vi "readFromXML.vi"(8 "error in (no error)":errorcluster, 10 "XML in":string, 11 "CableWrapCommands in":refnum<class "CableWrapCommands.lvclass">) -> (0 "error out":errorcluster, 3 "CableWrapCommands out":refnum<class "CableWrapCommands.lvclass">)   [LabVIEW 2014, in "TCSDataDefinitions.lvlib" / "TCSCommand.lvlib" / "CableWrapCommands.lvlib" / "CableWrapCommands.lvclass"]
uses:
  CableWrapCommands.lvclass
  CableWrapCommands.lvclass/CableWrapCommands.ctl
  TCSTcsCommand/TCSTcsCommand.lvclass
  <userlib>/Common/XML/XMLParser/XMLParser.lvclass
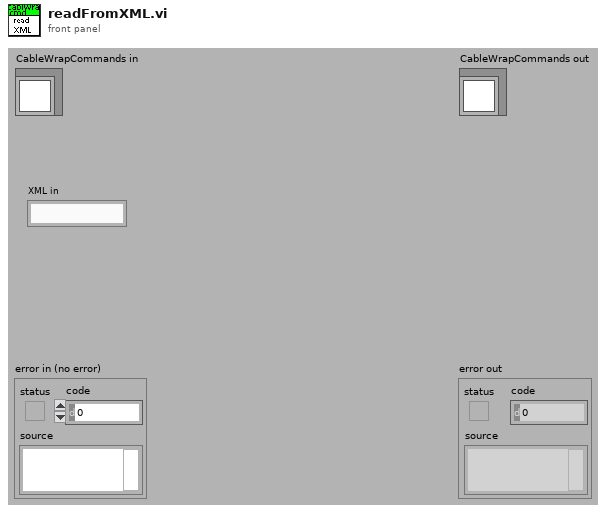
[diagram p1: front panel]
types:
  T1 = typedef "TCSDataDefinitions.lvlib/TCSCommand.lvlib/CableWrapCommands.lvlib/WrapnumTypes.ctl" = enum16{"-1", "0", "1"}
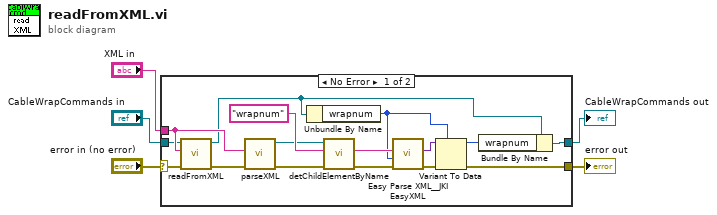
[diagram p0: block diagram]
diagram:
  n1 = case shown="No Error" "error in (no error)" {
    selector: "error in (no error)" -> [w21 w23]
    tunnel: [w9 w23] -> w4
    tunnel: [w14 w22] -> w2
    tunnel: "CableWrapCommands in" -> [w18 w22]
    tunnel: "XML in" -> [w20 _]
    frame No Error {
      n2 = call-parent "readFromXML.vi"("error in (no error)"=w21, "XMLin"=w20, "TCSTcsCommand in"=w18) -> ("error out"=w19:errorcluster, "TCSTcsCommand out"=w15:refnum<class "CableWrapCommands.lvclass">)  [unwired: 7 out]
      n3 = call <userlib>:"parseXML.vi"("error in (no error)"=w19, "XMLString in"=w20) -> ("error out"=w16:errorcluster, "Element out"=w6:refnum<class "XMLParser.lvclass">)  [unwired: 8 in]
      n4 = Unbundle By Name(w15) -> ("wrapnum"=w8:T1)
      n5 = call <userlib>:"detChildElementByName.vi"("error in (no error)"=w16, "childName"="wrapnum" ("ChildName"), "Element in"=w6) -> ("error out"=w12:errorcluster, "childXML"=w13:string)  [unwired: 5 in, 2 out]
      n6 = call <vilib>:"Easy Parse XML__JKI EasyXML.vi"("error in (no error)"=w12, "LabVIEW Data (Type)"=w8, "XML String"=w13) -> ("error out"=w10:errorcluster, "LabVIEW Data"=w11:variant)  [unwired: 7 in]
      n7 = Variant To Data(error in=w10, type=w8, Variant=w11) -> (data=w7:T1, error out=w9:errorcluster)
      n8 = Bundle By Name(cluster=w15, "wrapnum"=w7) -> (w14:refnum<class "CableWrapCommands.lvclass">)
    }
    frame Error {
    }
  }
  "error out" <- w4
  "CableWrapCommands out" <- w2
